vi "4110_Config.vi"(8 "error in (no error)":errorcluster, 10 "Specified Channel Ref List":T2[](array[typedef]) format="%.0x", 11 "Device Ref out":T2 format="%.0x") -> (0 "error out":errorcluster, 2 "Channel Info":T1(array[cluster]), 3 "Channel Ref List (out)":T2[](array[typedef]) format="%.0x")   [LabVIEW 2015, in "NI PXI-4110 Programmable Power Supply Custom Device.lvlib"]
uses:
  NI PXI-4110 Programmable Power Supply Custom Device.lvlib
  <vilib>/NI Veristand/Custom Device API/Custom Device Item Ref.ctl
  <instrlib>/niDCPower/nidcpower.llb/niDCPower Output Function.ctl
  4110_Global.vi
  <vilib>/NI Veristand/Custom Device API/Get Item Property (String).vi
  <vilib>/NI Veristand/Custom Device API/Get Item Property (U16).vi
  <vilib>/NI Veristand/Custom Device API/Get Item Property (I32).vi
  <vilib>/NI Veristand/Custom Device API/Get Item Property (Double).vi
  <vilib>/NI VeriStand/Custom Device API/Custom Device API.lvlib
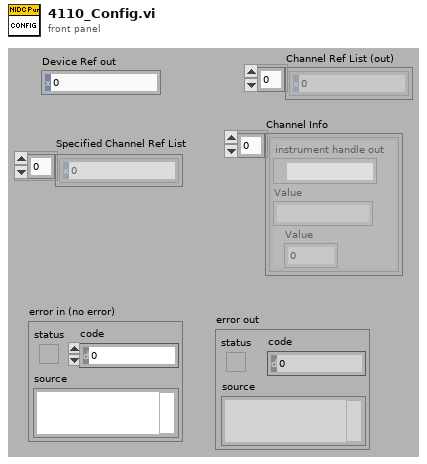
[diagram p1: front panel]
types:
  T1 = cluster{"instrument handle out":refnum<k15>, "Value":string, "Value":u16}[]
  T2 = typedef "Custom Device API.lvlib/Custom Device Item Ref.ctl" = u64
  T3 = typedef "niDCPower Output Function.ctl" = i32
  T4 = cluster{"instrument handle out":refnum<k15>, string, "Value":u16}
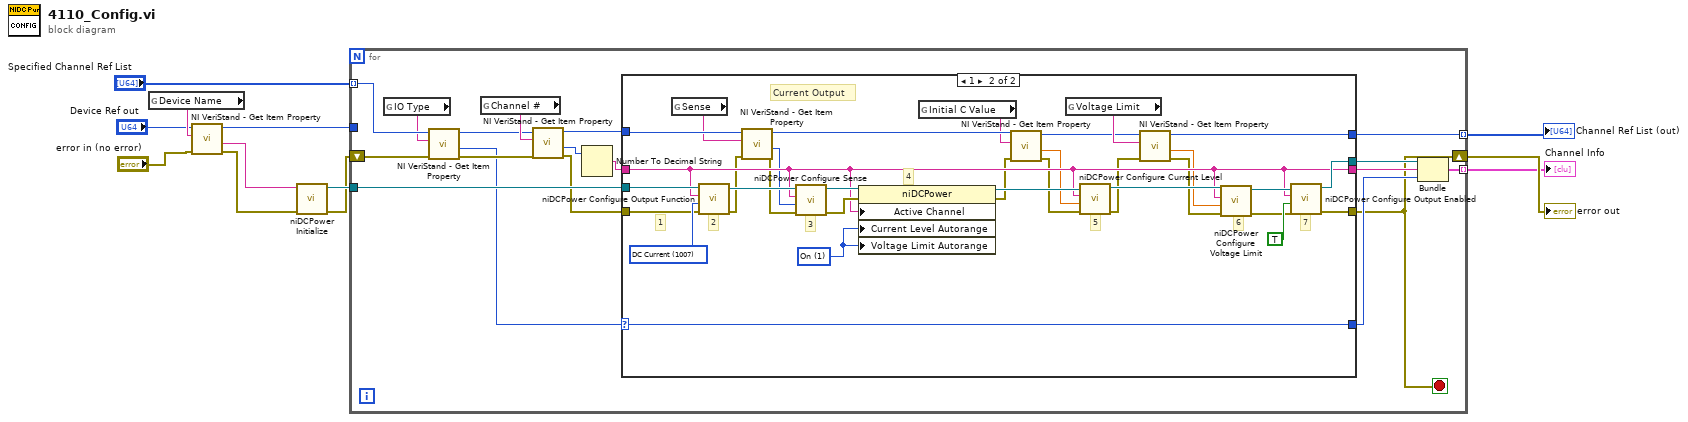
[diagram p0: block diagram]
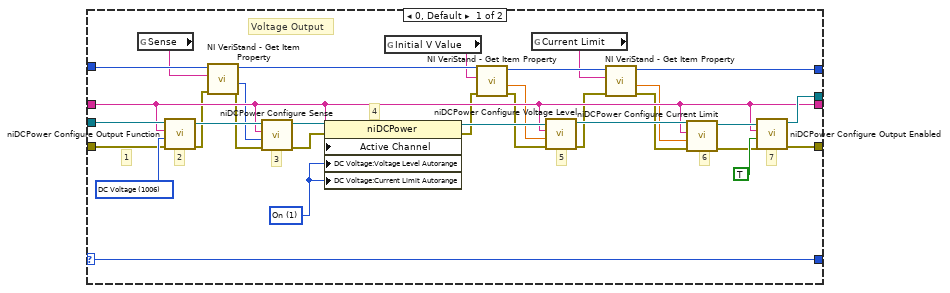
[diagram p2: hidden frame]
diagram:
  n1 = global read "4110_Global.vi" "Device Name"() -> (w10:string)
  n2 = call-poly <vilib>:"NI VeriStand - Get Item Property.vi"("error in (no error)"="error in (no error)", "Property Name"=w10, "Item Ref in"="Device Ref out") -> ("error out"=w7:errorcluster, "Value"=w1:string, "Item Ref out"=w6:T2)  [unwired: 5 in, 1 out]
  n3 = call <instrlib>:"niDCPower Initialize.vi"("error in (no error)"=w7, "resource name"=w1) -> ("error out"=w4:errorcluster, "instrument handle out"=w5:refnum<k15>)  [unwired: 2 in, 6 out]
  n4 = for {
    tunnel: "Specified Channel Ref List" -> [w26] mode=indexing
    tunnel: [w29] -> w2 mode=indexing
    tunnel: w6 -> [_]
    tunnel: w5 -> [w23]
    tunnel: [w17] -> w3 mode=indexing
    shift-right: [w13] -> w11
    shift-left: w4 -> [w24]
    stop <- w13 stop-if-true
    n5 = global read "4110_Global.vi" "IO Type"() -> (w25:string)
    n6 = call-poly <vilib>:"NI VeriStand - Get Item Property.vi"("error in (no error)"=w24, "Property Name"=w25, "Item Ref in"=w26) -> ("error out"=w21:errorcluster, "Value"=w19:u16, "Item Ref out"=w22:T2)  [unwired: 5 in, 1 out]
    n7 = global read "4110_Global.vi" "Channel #"() -> (w30:string)
    n8 = call-poly <vilib>:"NI VeriStand - Get Item Property.vi"("error in (no error)"=w21, "Property Name"=w30, "Item Ref in"=w22) -> ("error out"=w18:errorcluster, "Value"=w14:u16, "Item Ref out"=w20:T2)  [unwired: 5 in, 1 out]
    n9 = Number To Decimal String(number=w14) -> (decimal integer string=w15:string)  [unwired: 1 in]
    n10 = case shown="1" w19 {
      selector: w19 -> [w31 w66]
      tunnel: [w52 w85] -> w13
      tunnel: [w51 w84] -> w28
      tunnel: [w49 w82] -> w27
      tunnel: w23 -> [w50 w83]
      tunnel: w20 -> [w48 w81]
      tunnel: w15 -> [w49 w82]
      tunnel: w18 -> [w45 w78]
      tunnel: [w32 w67] -> w17
      tunnel: [w31 w66] -> w16
      frame 0, Default {
        w61 = T3 1006 items=["DC Voltage"=1006, "DC Current"=1007] ("output function")
        w62 = 1 items=["Off", "On"] ("DC Voltage:Voltage Level Autorange")
        # "Voltage Output"
        # "7"
        # "6"
        # "5"
        # "2"
        # "4"
        # "3"
        # "1"
        n11 = global read "4110_Global.vi" "Sense"() -> (w47:string)
        n12 = call <instrlib>:"niDCPower Configure Output Function.vi"("error in (no error)"=w45, "output function"=w61, "channel name"=w49, "instrument handle"=w50) -> ("error out"=w44:errorcluster, "instrument handle out"=w60:refnum<k15>)  [unwired: 6 out]
        n13 = call-poly <vilib>:"NI VeriStand - Get Item Property.vi"("error in (no error)"=w44, "Property Name"=w47, "Item Ref in"=w48) -> ("error out"=w43:errorcluster, "Value"=w46:i32, "Item Ref out"=w42:T2)  [unwired: 5 in, 1 out]
        n14 = call <instrlib>:"niDCPower Configure Sense.vi"("error in (no error)"=w43, "sense"=w46, "channel name"=w49, "instrument handle"=w60) -> ("error out"=w59:errorcluster, "instrument handle out"=w53:refnum<k15>)  [unwired: 6 out]
        n15 = property class="niDCPower"(reference=w53, error in=w59, "Active Channel"=w49, "DC Voltage:Voltage Level Autorange"=w62, "DC Voltage:Current Limit Autorange"=w62) -> (reference out=w58:refnum<k15>, error out=w40:errorcluster)
        n16 = global read "4110_Global.vi" "Initial V Value"() -> (w41:string)
        n17 = call-poly <vilib>:"NI VeriStand - Get Item Property.vi"("error in (no error)"=w40, "Property Name"=w41, "Item Ref in"=w42) -> ("error out"=w39:errorcluster, "Value"=w38:dbl, "Item Ref out"=w37:T2)  [unwired: 5 in, 1 out]
        n18 = global read "4110_Global.vi" "Current Limit"() -> (w36:string)
        n19 = call <instrlib>:"niDCPower Configure Voltage Level.vi"("error in (no error)"=w39, "voltage level"=w38, "channel name"=w49, "instrument handle"=w58) -> ("error out"=w35:errorcluster, "instrument handle out"=w56:refnum<k15>)  [unwired: 6 out]
        n20 = call-poly <vilib>:"NI VeriStand - Get Item Property.vi"("error in (no error)"=w35, "Property Name"=w36, "Item Ref in"=w37) -> ("error out"=w34:errorcluster, "Value"=w33:dbl, "Item Ref out"=w32:T2)  [unwired: 5 in, 1 out]
        n21 = call <instrlib>:"niDCPower Configure Current Limit.vi"("error in (no error)"=w34, "current limit"=w33, "channel name"=w49, "instrument handle"=w56) -> ("error out"=w54:errorcluster, "instrument handle out"=w55:refnum<k15>)  [unwired: 1 in, 5 out]
        n22 = call <instrlib>:"niDCPower Configure Output Enabled.vi"("error in (no error)"=w54, "output enabled"=TRUE ("Output Enabled"), "channel name"=w49, "instrument handle"=w55) -> ("error out"=w52:errorcluster, "instrument handle out"=w51:refnum<k15>)  [unwired: 6 out]
      }
      frame 1 {
        w94 = T3 1007 items=["DC Voltage"=1006, "DC Current"=1007] ("output function")
        w63 = 1 items=["Off", "On"] ("DC Voltage:Voltage Level Autorange")
        # "Current Output"
        # "7"
        # "6"
        # "5"
        # "2"
        # "4"
        # "3"
        # "1"
        n23 = global read "4110_Global.vi" "Sense"() -> (w80:string)
        n24 = call <instrlib>:"niDCPower Configure Output Function.vi"("error in (no error)"=w78, "output function"=w94, "channel name"=w82, "instrument handle"=w83) -> ("error out"=w77:errorcluster, "instrument handle out"=w93:refnum<k15>)  [unwired: 6 out]
        n25 = call-poly <vilib>:"NI VeriStand - Get Item Property.vi"("error in (no error)"=w77, "Property Name"=w80, "Item Ref in"=w81) -> ("error out"=w76:errorcluster, "Value"=w79:i32, "Item Ref out"=w75:T2)  [unwired: 5 in, 1 out]
        n26 = call <instrlib>:"niDCPower Configure Sense.vi"("error in (no error)"=w76, "sense"=w79, "channel name"=w82, "instrument handle"=w93) -> ("error out"=w92:errorcluster, "instrument handle out"=w86:refnum<k15>)  [unwired: 6 out]
        n27 = property class="niDCPower"(reference=w86, error in=w92, "Active Channel"=w82, "Current Level Autorange"=w63, "Voltage Limit Autorange"=w63) -> (reference out=w91:refnum<k15>, error out=w73:errorcluster)
        n28 = global read "4110_Global.vi" "Initial C Value"() -> (w74:string)
        n29 = call-poly <vilib>:"NI VeriStand - Get Item Property.vi"("error in (no error)"=w73, "Property Name"=w74, "Item Ref in"=w75) -> ("error out"=w72:errorcluster, "Value"=w64:dbl, "Item Ref out"=w65:T2)  [unwired: 5 in, 1 out]
        n30 = global read "4110_Global.vi" "Voltage Limit"() -> (w71:string)
        n31 = call <instrlib>:"niDCPower Configure Current Level.vi"("error in (no error)"=w72, "current level"=w64, "channel name"=w82, "instrument handle"=w91) -> ("error out"=w70:errorcluster, "instrument handle out"=w89:refnum<k15>)  [unwired: 6 in]
        n32 = call-poly <vilib>:"NI VeriStand - Get Item Property.vi"("error in (no error)"=w70, "Property Name"=w71, "Item Ref in"=w65) -> ("error out"=w69:errorcluster, "Value"=w68:dbl, "Item Ref out"=w67:T2)  [unwired: 5 in, 1 out]
        n33 = call <instrlib>:"niDCPower Configure Voltage Limit.vi"("error in (no error)"=w69, "voltage limit"=w68, "channel name"=w82, "instrument handle"=w89) -> ("error out"=w87:errorcluster, "instrument handle out"=w88:refnum<k15>)  [unwired: 6 in]
        n34 = call <instrlib>:"niDCPower Configure Output Enabled.vi"("error in (no error)"=w87, "output enabled"=TRUE ("Output Enabled"), "channel name"=w82, "instrument handle"=w88) -> ("error out"=w85:errorcluster, "instrument handle out"=w84:refnum<k15>)  [unwired: 6 out]
      }
    }
    n35 = Bundle("instrument handle out"=w28, w27, "Value"=w16) -> (w29:T4)  [unwired: 1 in]
  }
  "error out" <- w11
  "Channel Ref List (out)" <- w3
  "Channel Info" <- w2
